vi "close motor.vi"(8 "error in (no error)":errorcluster, 11 ".NET Refnum in":refnum<k24>) -> ()   [LabVIEW 2017]
uses:
  Newport.CONEXCC.CommandInterface
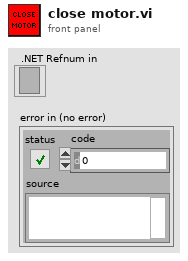
[diagram p1: front panel]
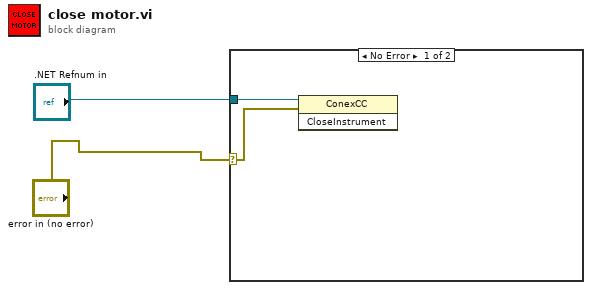
[diagram p0: block diagram]
diagram:
  n1 = case shown="No Error" "error in (no error)" {
    selector: "error in (no error)" -> [w3 _]
    tunnel: ".NET Refnum in" -> [w4 _]
    frame No Error {
      n2 = invoke class="ConexCC" method="CloseInstrument"(reference=w4, error in=w3) -> ()  [unwired: 1 in, 3 out]
    }
    frame Error {
    }
  }
